vi "DeltaX.vi"(1 "Array in":dbl[](array[numeric])) -> (0 "Array out":dbl[](array[numeric]))   [LabVIEW 2017]
doc: "Calcula la diferencia entre los elementos de un vector"
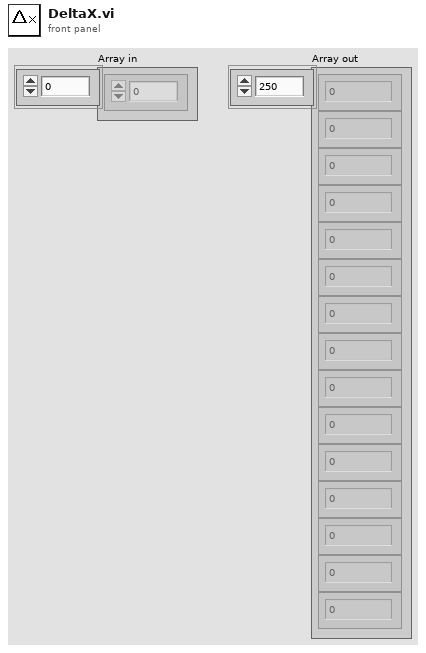
[diagram p1: front panel]
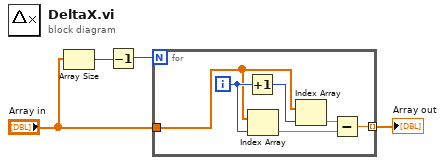
[diagram p0: block diagram]
diagram:
  n1 = Array Size(array="Array in") -> (size(s)=w1:i32)
  n2 = Decrement(x=w1) -> (x-1=w2:i32)
  n3 = for {
    N: w2 -> [_]
    tunnel: "Array in" -> [w8]
    tunnel: [w5] -> w3 mode=indexing
    i -> [w9]
    n4 = Increment(x=w9) -> (x+1=w10:i32)
    n5 = Index Array(array=w8, index=w9) -> (element=w6:dbl)
    n6 = Index Array(array=w8, index=w10) -> (element=w7:dbl)
    n7 = Subtract(x=w7, y=w6) -> (x-y=w5:dbl)
  }
  "Array out" <- w3
